vi "Sequencer Main.vi"() -> ()   [LabVIEW 2018] (continued)
                    }
                  }
                  n3171 = call <userlib>:"Clear All Errors__ogtk.vi"("Error In"=w6450) -> ()  [unwired: 3 in, 1 out]
                }
              }
            }
            frame #5 {
              n3172 = in-place {
                n3173 = local read "Gen Test Status"() -> (w6474:bool)
                n3174 = local read "Cnt Total All"() -> (w6475:i32)
                n3175 = case shown="False" w6474 {
                  frame False {
                    n3176 = local read "Cnt False All"() -> (w6477:i32)
                    n3177 = Increment(x=w6477) -> (x+1=w6478:i32)
                    n3178 = local write "Cnt False All"(w6478) -> ()
                  }
                  frame True {
                    n3179 = local read "Cnt Pass All"() -> (w6479:i32)
                    n3180 = Increment(x=w6479) -> (x+1=w6480:i32)
                    n3181 = local write "Cnt Pass All"(w6480) -> ()
                  }
                }
                n3182 = Increment(x=w6475) -> (x+1=w6476:i32)
                n3183 = local write "Cnt Total All"(w6476) -> ()
              }
              n3184 = global write "Global Variable.vi" "System Status"(T1."Idle" ("System Status")) -> ()
              n3185 = property on="Tab Control Main" class="TabCtl (strict)"("Value"=T2."TEST Board" ("Tab Control Main")) -> ()  [unwired: 2 in, 2 out]
            }
            frame #6 {
              n3186 = local read "System INI Config File"() -> (w6481:path)
              n3187 = in-place {
                in-place-border: w6481 -> [w6493]
                w6494 = "REPORT"
                # "Write DATA To INI Sys File"
                n3188 = local read "Cnt Total All"() -> (w6489:i32)
                n3189 = call <vilib>:"Open Config Data.vi"("configuration file path"=w6493) -> ("error out"=w6491:errorcluster, "refnum"=w6492:T19)  [unwired: 8 in, 1 out]
                n3190 = local read "Cnt Pass All"() -> (w6482:i32)
                n3191 = call-poly <vilib>:"Write Key.vi"("section"=w6494, "error in (no error)"=w6491, "value"=w6489, "key"="TOTAL", "refnum"=w6492) -> ("error out"=w6495:errorcluster, "refnum out"=w6498:T19)  [unwired: 4 in, 1 out]
                n3192 = local read "Cnt False All"() -> (w6483:i32)
                n3193 = call-poly <vilib>:"Write Key.vi"("section"=w6494, "error in (no error)"=w6495, "value"=w6482, "key"="PASS", "refnum"=w6498) -> ("error out"=w6496:errorcluster, "refnum out"=w6497:T19)  [unwired: 4 in, 1 out]
                n3194 = call-poly <vilib>:"Write Key.vi"("section"=w6494, "error in (no error)"=w6496, "value"=w6483, "key"="FALSE", "refnum"=w6497) -> ("error out"=w6485:errorcluster, "refnum out"=w6486:T19)  [unwired: 4 in, 1 out]
                n3195 = call <vilib>:"Close Config Data.vi"("error in (no error)"=w6485, "refnum"=w6486) -> ("error out"=w6484:errorcluster)  [unwired: 8 in, 1 out]
                n3196 = call <vilib>:"Simple Error Handler.vi"("error in (no error)"=w6484) -> ()  [unwired: 4 in, 5 out]
              }
            }
          }
        }
        frame "QUIT" {
        }
        frame "Test Load Monitor" {
          n3197 = global write "Global Variable.vi" "System Status"(T1."Idle" ("System Status")) -> ()
        }
      }
    }
  }
